vi "Get SMO Port.vi"(8 "error in (no error)":errorcluster, 11 "ExampleInstrument in":refnum<class "Instrument.LN2.lvclass">) -> (0 "error out":errorcluster, 2 "Port":u16, 3 "ExampleInstrument out":refnum<class "Instrument.LN2.lvclass">)   [LabVIEW 2019, in "Instrument.LN2.lvclass"]
uses:
  Instrument.LN2.lvclass
  <userlib>/LevyLab/Instrument Framework/Instrument Types/VSource/Instrument.VSource.lvclass
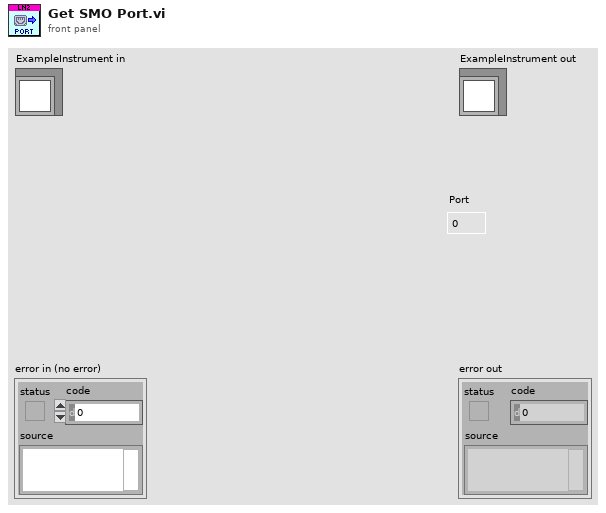
[diagram p1: front panel]
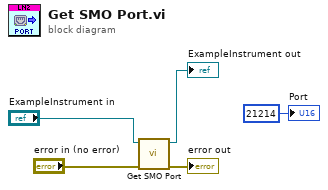
[diagram p0: block diagram]
diagram:
  n1 = call-parent "Get SMO Port.vi"("error in (no error)"="error in (no error)", "Instrument in"="ExampleInstrument in") -> ("error out"=→"error out":errorcluster, "Instrument out"=→"ExampleInstrument out":refnum<class "Instrument.LN2.lvclass">)  [unwired: 7 in, 1 out]
  "Port" <- u16 21214 ("Port")
